vi "Fit Circle - 2D.vi"(8 "error in (no error)":errorcluster, 11 "Points":refnum<class "Vec3d.lvclass">[](array[class])) -> (0 "error out":errorcluster, 1 "Residual":dbl, 2 "Radius":dbl, 3 "Center":refnum<class "Vec3d.lvclass">)   [LabVIEW 2023]
uses:
  Vec3d Class/Vec3d.lvclass
  <vilib>/Analysis/baseanly.llb/Mean (DBL).vi
  <vilib>/Analysis/baseanly.llb/Real A x B.vi
  <vilib>/Analysis/baseanly.llb/Real Inverse Matrix.vi
  <vilib>/Analysis/NI_AALBase.lvlib
panel:
  out "Center":cluster{"X":dbl, "Y":dbl, "Z":dbl}
  out "Fit Results":cluster{"Xs":dbl[], "Ys":dbl[]}[](graph)
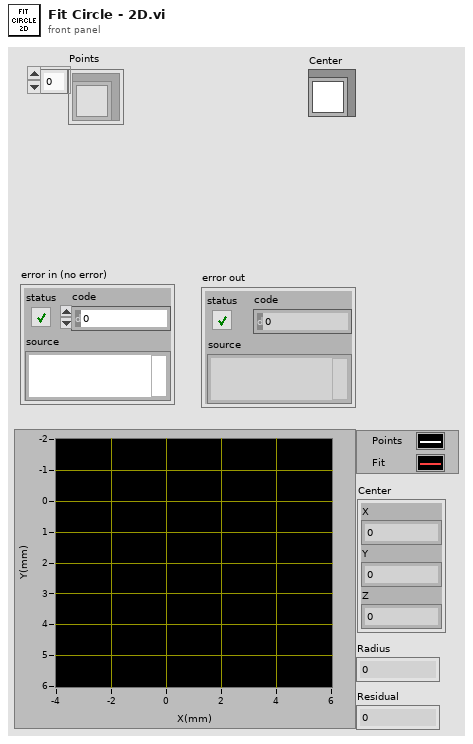
[diagram p1: front panel]
types:
  T1 = typedef "NI_Matrix.lvlib/RealMatrix.ctl" = dbl[][]
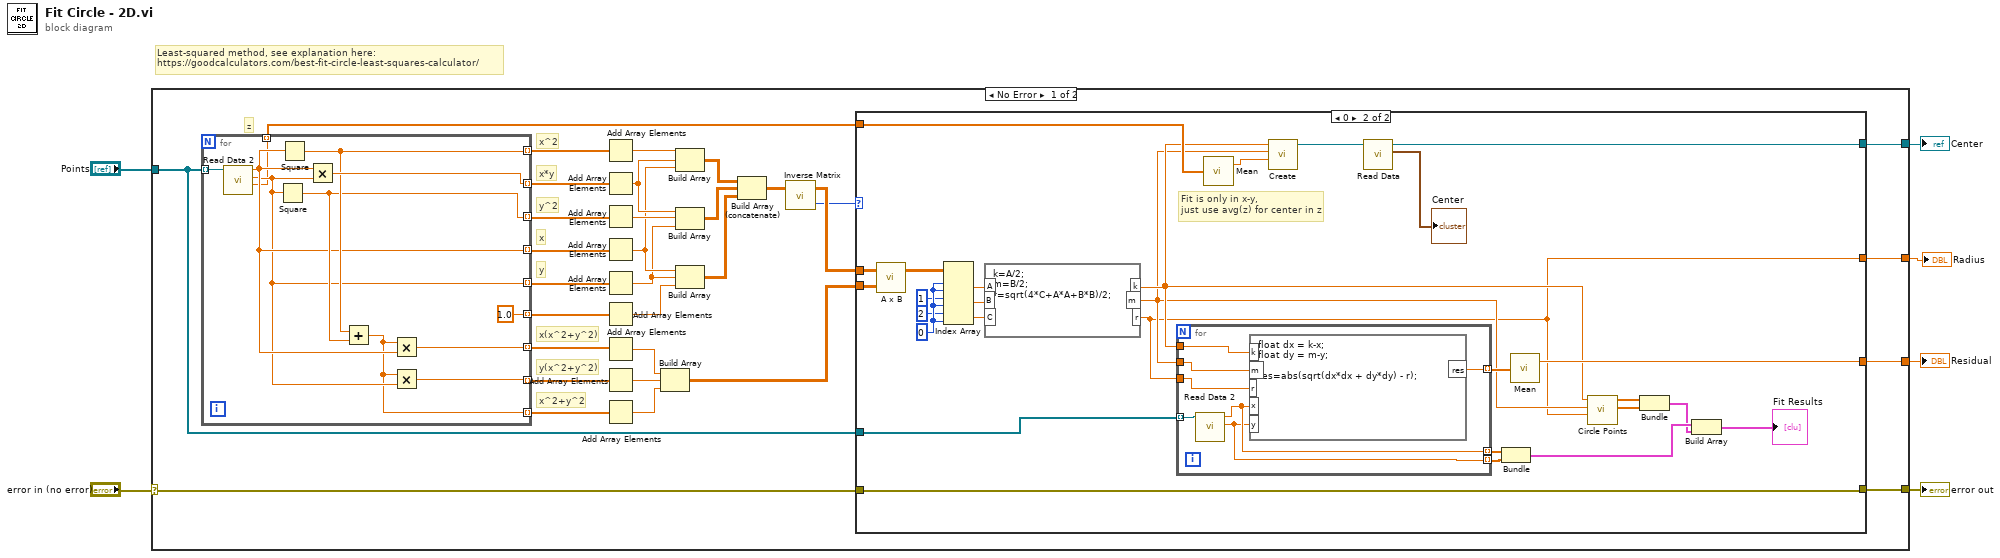
[diagram p0: block diagram]
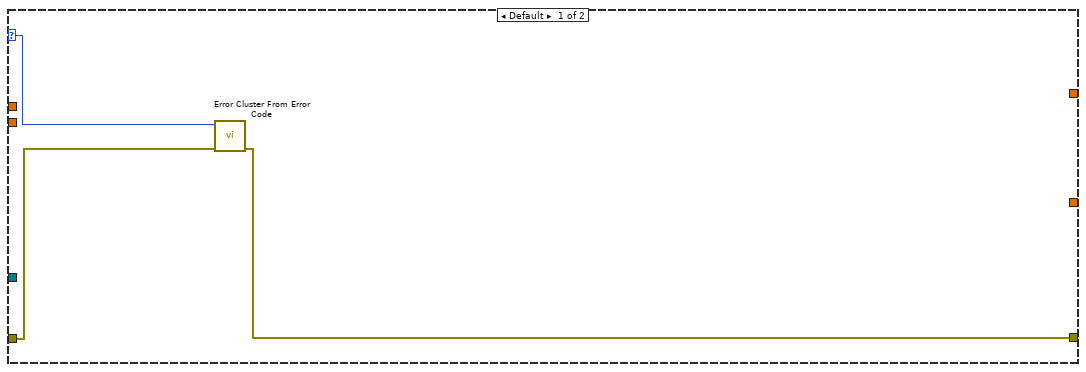
[diagram p2: hidden frame]
diagram:
  # "Least-squared method, see explanation here:\nhttps://goodcalculators.com/best-fit-circle-least-squares-calculator/"
  n1 = case shown="No Error" "error in (no error)" {
    selector: "error in (no error)" -> [w8 w88]
    tunnel: "Points" -> [w14 _]
    tunnel: [w13 _] -> w4
    tunnel: [w11 _] -> w3
    tunnel: [w9 _] -> w2
    tunnel: [w7 w88] -> w1
    frame No Error {
      # "z"
      # "x^2+y^2"
      # "y(x^2+y^2)"
      # "x(x^2+y^2)"
      # "y"
      # "x"
      # "y^2"
      # "x*y"
      # "x^2"
      n2 = for {
        tunnel: w14 -> [w87] mode=indexing
        tunnel: [w84] -> w38 mode=indexing
        tunnel: [w86] -> w35 mode=indexing
        tunnel: [w83] -> w34 mode=indexing
        tunnel: [w82] -> w33 mode=indexing
        tunnel: [w80] -> w36 mode=indexing
        tunnel: [1.0] -> w37 mode=indexing
        tunnel: [w81] -> w22 mode=indexing
        tunnel: [w79] -> w21 mode=indexing
        tunnel: [w78] -> w20 mode=indexing
        tunnel: [w77] -> w12 mode=indexing
        n3 = call-dynamic "Read Data 2.vi"("Vec3d in"=w87) -> ("Z"=w77:dbl, "Y"=w80:dbl, "X"=w82:dbl)  [unwired: 7 in, 1 out]
        n4 = Square(x=w80) -> (x^2=w83:dbl)
        n5 = Square(x=w82) -> (x^2=w84:dbl)
        n6 = Multiply(x=w82, y=w80) -> (x*y=w86:dbl)
        n7 = Add(x=w84, y=w83) -> (x+y=w78:dbl)
        n8 = Multiply(x=w78, y=w82) -> (x*y=w81:dbl)
        n9 = Multiply(x=w78, y=w80) -> (x*y=w79:dbl)
      }
      n10 = Add Array Elements(numeric array=w38) -> (sum=w32:dbl)
      n11 = Add Array Elements(numeric array=w35) -> (sum=w31:dbl)
      n12 = Add Array Elements(numeric array=w34) -> (sum=w30:dbl)
      n13 = Add Array Elements(numeric array=w33) -> (sum=w29:dbl)
      n14 = Add Array Elements(numeric array=w36) -> (sum=w28:dbl)
      n15 = Add Array Elements(numeric array=w37) -> (sum=w27:dbl)
      n16 = Add Array Elements(numeric array=w22) -> (sum=w19:dbl)
      n17 = Add Array Elements(numeric array=w21) -> (sum=w18:dbl)
      n18 = Add Array Elements(numeric array=w20) -> (sum=w17:dbl)
      n19 = Build Array(w19, w18, w17) -> (w15:T1)
      n20 = Build Array(w32, w31, w29) -> (w26:T1)
      n21 = Build Array(w31, w30, w28) -> (w25:T1)
      n22 = Build Array(w29, w28, w27) -> (w24:T1)
      n23 = Build Array (concatenate)(w26, w25, w24) -> (w23:T1)
      n24 = call-poly <vilib>:"Inverse Matrix.vi"("Input Matrix"=w23) -> ("error"=w10:i32, "Inverse Matrix"=w16:T1)  [unwired: 1 in]
      n25 = case shown="0" w10 {
        selector: w10 -> [w41 _]
        tunnel: w16 -> [_ w69]
        tunnel: w15 -> [_ w68]
        tunnel: w14 -> [_ w60]
        tunnel: [_ w58] -> w13
        tunnel: w12 -> [_ w57]
        tunnel: [_ w53] -> w11
        tunnel: [_ w49] -> w9
        tunnel: w8 -> [w40 w55]
        tunnel: [w39 w55] -> w7
        frame Default {
          n26 = call <vilib>:"Error Cluster From Error Code.vi"("error in (no error)"=w40, "error code (0)"=w41) -> ("error out"=w39:errorcluster)  [unwired: 7 in]
        }
        frame 0 {
          w66 = 0 ("index (row)")
          # "Fit is only in x-y, \njust use avg(z) for center in z"
          n27 = call-poly <vilib>:"A x B.vi"("B"=w68, "A"=w69) -> ("A x B"=w67:T1)  [unwired: 1 out]
          n28 = Index Array(array=w67, index (row) #1=w66, index (col) #1=w66, index (row) #2=1 ("index (row)"), index (col) #2=w66, index (row) #3=2 ("index (row)"), index (col) #3=w66) -> (element #1=w63:dbl, element #2=w62:dbl, element #3=w61:dbl)
          n29 = formula code="k=A/2;\nm=B/2;\nr=sqrt(4*C+A*A+B*B)/2;"("A"=w63, "B"=w62, "C"=w61) -> ("k"=w51:dbl, "m"=w50:dbl, "r"=w49:dbl)
          n30 = for {
            tunnel: w60 -> [w76] mode=indexing
            tunnel: w51 -> [w75]
            tunnel: w50 -> [w74]
            tunnel: w49 -> [w73]
            tunnel: [w72] -> w59 mode=indexing
            tunnel: [w71] -> w46 mode=indexing
            tunnel: [w70] -> w45 mode=indexing
            n31 = call-dynamic "Read Data 2.vi"("Vec3d in"=w76) -> ("Y"=w70:dbl, "X"=w71:dbl)  [unwired: 7 in, 2 out]
            n32 = formula code="float dx = k-x;\nfloat dy = m-y;\n\nres=abs(sqrt(dx*dx + dy*dy) - r);"("k"=w75, "m"=w74, "r"=w73, "x"=w71, "y"=w70) -> ("res"=w72:dbl)
          }
          n33 = call-poly <vilib>:"Mean.vi"("X"=w57) -> ("mean"=w56:dbl)  [unwired: 1 out]
          n34 = call "Create.vi"("Z"=w56, "Y"=w50, "X"=w51) -> ("Vec3d Class out"=w54:refnum<class "Vec3d.lvclass">)  [unwired: 7 in, 1 out]
          n35 = call-dynamic "Read Data.vi"("Vec3d Class in"=w54) -> ("Data"=→"Center":cluster{"X":dbl, "Y":dbl, "Z":dbl}, "Vec3d Class out"=w53:refnum<class "Vec3d.lvclass">)  [unwired: 8 in, 1 out]
          n36 = Bundle(w46, w45) -> (w44:cluster{dbl[], dbl[]})  [unwired: 1 in]
          n37 = call-poly <vilib>:"Mean.vi"("X"=w59) -> ("mean"=w58:dbl)  [unwired: 1 out]
          n38 = call "Circle Points.vi"("Radius"=w49, "Y"=w50, "X"=w51) -> ("Ys"=w47:dbl[], "Xs"=w48:dbl[])  [unwired: 7 in]
          n39 = Bundle("Xs"=w48, "Ys"=w47) -> (w43:cluster{"Xs":dbl[], "Ys":dbl[]})  [unwired: 1 in]
          n40 = Build Array(w44, w43) -> (→"Fit Results":cluster{"Xs":dbl[], "Ys":dbl[]}[])
        }
      }
    }
    frame Error {
    }
  }
  "Center" <- w3
  "Residual" <- w4
  "error out" <- w1
  "Radius" <- w2
